vi "Reverse StartDelay.vi"(0 "Start Delay":dbl[](array[numeric]), 5 "Relative To":T1[](array[typedef]) items=["Power sequence start", "Previous source start", "Previous source end"]) -> (4 "Start Delay OUT":dbl[](array[numeric]), 6 "Relative To OUT":T1[](array[typedef]) items=["Power sequence start", "Previous source start", "Previous source end"])   [LabVIEW 2024, in "devicePowerSequencerCoreLogic.lvlib"]
uses:
  devicePowerSequencerCoreLogic.lvlib
  controls/Relative To.ctl
  devicePowerSequencer.lvlib
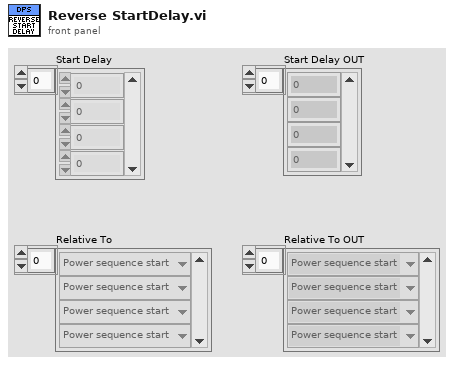
[diagram p1: front panel]
types:
  T1 = typedef "devicePowerSequencer.lvlib/Relative To.ctl" = u32
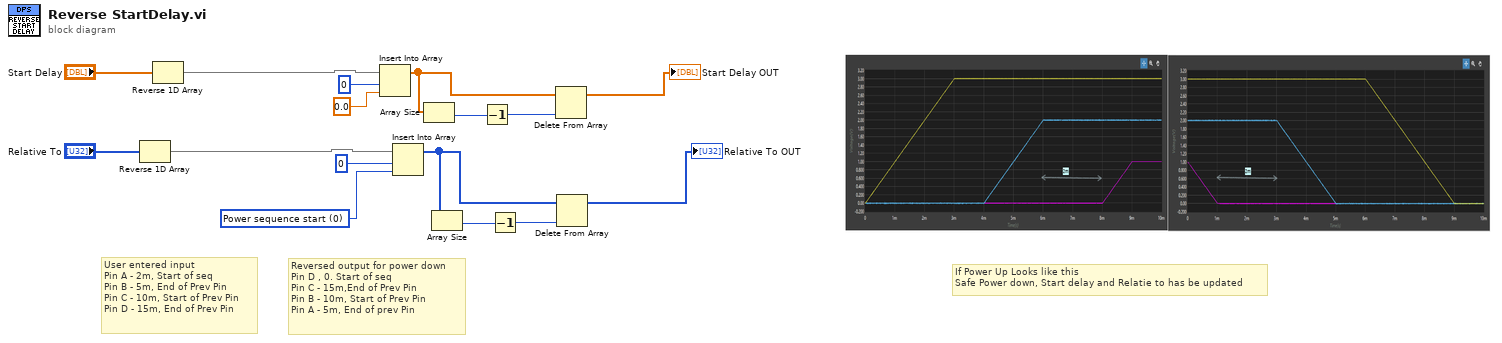
[diagram p0: block diagram]
diagram:
  w12 = T1 0 items=["Power sequence start", "Previous source start", "Previous source end"] ("new element/subarray")
  # "Reversed output for power down\nPin D , 0. Start of seq\nPin C - 15m,End of Prev Pin\nPin B - 10m, Start of Prev Pin\nPin A - 5m, End of prev Pin"
  # "User entered input\nPin A - 2m, Start of seq\nPin B - 5m, End of Prev Pin\nPin C - 10m, Start of Prev Pin\nPin D - 15m, End of Prev Pin"
  # "If Power Up Looks like this\nSafe Power down, Start delay and Relatie to has be updated"
  n1 = Reverse 1D Array(array="Relative To") -> (reversed array=w10:T1[])
  n2 = Reverse 1D Array(array="Start Delay") -> (reversed array=w11:dbl[])
  n3 = Insert Into Array(array=w11, index=0, new element=0.0 ("new element/subarray")) -> (w9:dbl[])
  n4 = Insert Into Array(array=w10, index=0, new element=w12) -> (w5:T1[])
  n5 = Array Size(array=w9) -> (size(s)=w8:i32)
  n6 = Array Size(array=w5) -> (size(s)=w6:i32)
  n7 = Decrement(x=w8) -> (x-1=w2:i32)
  n8 = Decrement(x=w6) -> (x-1=w7:i32)
  n9 = Delete From Array(array=w9, index=w2) -> (array with subset deleted=→"Start Delay OUT":dbl[])  [unwired: 1 in, 1 out]
  n10 = Delete From Array(array=w5, index=w7) -> (array with subset deleted=→"Relative To OUT":T1[])  [unwired: 1 in, 1 out]
